vi "SwTmr Main.vi"() -> ()   [LabVIEW 2017]
doc: "This sample project is built upon the standard state machine template and shows how you could create an application that acquires, analyzes, and presents data. It includes functionality for presenting configuration dialogs, preserving settings between executions, loading and saving data, as well as exporting graph images and text files.\n\nIt is most appropriate for data that is acquired instantly as it does not allow for screen updates mid acquisition nor does it allow for continuous streaming to disk."
uses:
  controls/SwTmr State.ctl
  controls/SwTmr Data.ctl
  controls/SwTmr UI References.ctl
  controls/SwTmr Graph Data.ctl
  <vilib>/Utility/miscctls.llb/LVAnnotationListTypeDef.ctl
  <vilib>/Utility/miscctls.llb/LVCursorListTypeDef.ctl
  controls/SwTmr User Specified Data.ctl
  controls/SwTmr HW Configuration.ctl
  controls/SwTmr Analysis Configuration.ctl
  controls/SwTmr New Data Behavior.ctl
  controls/SwTmr Transfer Func File Path.ctl
  <vilib>/Utility/file.llb/Read Delimited Spreadsheet (DBL).vi
panel:
  in  "Settings":bool
  in  "Snapshot":bool
  in  "Analyze":bool
  in  "Clear":bool
  in  "Exit":bool
  in  "Acquire":bool
  in  "Export":bool
  in  "Save Data":bool
  in  "Load Data":bool
  out "Ch4 Error (mm:ss)":dbl format="%<%M:%S>t"
  out "Ch3 Error (mm:ss)":dbl format="%<%M:%S>t"
  out "Ch2 Error (mm:ss)":dbl format="%<%M:%S>t"
  out "Ch1 Error (mm:ss)":dbl format="%<%M:%S>t"
  out "Ch0 Error (mm:ss)":dbl format="%<%M:%S>t"
  out "Ch4 Time (mm:ss)":dbl format="%<%M:%S>t"
  out "Ch3 Time (mm:ss)":dbl format="%<%M:%S>t"
  out "Ch2 Time (mm:ss)":dbl format="%<%M:%S>t"
  out "Ch1 Time (mm:ss)":dbl format="%<%M:%S>t"
  out "Ch0 Time (mm:ss)":dbl format="%<%M:%S>t"
  out "Raw Data Graph":waveform(dbl)[](graph)
  out "Status Bar":string
  # "ROGERS RESEARCH GROUP"
  # "Electrochemical Stopwatch Readout System"
  # "+/-"
  # "+/-"
  # "+/-"
  # "+/-"
  # "+/-"
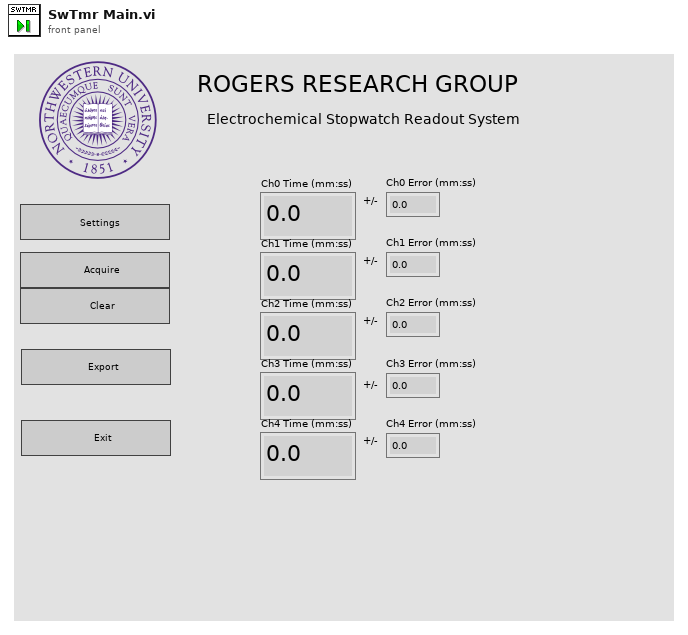
[diagram p1: front panel]
types:
  T1 = typedef "SwTmr Data.ctl" = cluster{"UI References":T2, "Graph Data":T3, "User Specified":T6}
  T2 = typedef "SwTmr UI References.ctl" = cluster{"Stop Ref":refnum<vi>, "Save Ref":refnum<vi>, "Open Ref":refnum<vi>, "Export Ref":refnum<vi>, "Acquire Ref":refnum<vi>, "Configure Ref":refnum<vi>, "Graph Ref":refnum<vi>, "Clear Ref":refnum<vi>, "Analyze Ref":refnum<vi>, "Status Ref":refnum<vi>, "Snapshot Ref":refnum<vi>}
  T3 = typedef "SwTmr Graph Data.ctl" = cluster{"Data":waveform(dbl)[], "Annotation List":T4, "Cursor List":T5, "Analysis Data":waveform(dbl)[]}
  T4 = typedef "LVAnnotationListTypeDef.ctl" = cluster{"Name":string, "Color":u32, "Style":u8, "Point Style":u8, "Name Visible":bool, "Allow Drag":bool, "Annotation Mode":u32, "Plot":i32, "Index":i32, "Position":cluster{"X":dbl, "Y":dbl}, "X Scale":u32, "Y Scale":u32, "Show Arrow":bool, "Lock Name":bool, "Plot Area":i32, "Label Offset":cluster{"X":dbl, "Y":dbl}}[]
  T5 = typedef "LVCursorListTypeDef.ctl" = cluster{"Name":string, "Color":u32, "Style":u8, "Point Style":u8, "Name Visible":bool, "Allow Drag":bool, "Cursor Mode":u32, "Plot":i32, "Index":i32, "Position":cluster{"X":dbl, "Y":dbl}, "X Scale":u32, "Y Scale":u32, "Watch Plots":i32[], "Watch All Plots":bool, "Plot Area":i32, "Label Offset":cluster{"X":dbl, "Y":dbl}}[]
  T6 = typedef "SwTmr User Specified Data.ctl" = cluster{"Hardware Configuration":T7, "Analysis Configuration":T8, "New Data Behavior":T9, "Time-Voltage transfer function file path (dialog if empty)":T10, "Cell (V) Error Upper":dbl, "Cell (V) Error Lower (type \"-\")":dbl}
  T7 = typedef "SwTmr HW Configuration.ctl" = cluster{"Physical Channel":tag, "Maximum Input":dbl, "Minimum Input":dbl, "Sample Rate":dbl, "Number of Samples":i32}
  T8 = typedef "SwTmr Analysis Configuration.ctl" = cluster{"Statistics":bool}
  T9 = typedef "SwTmr New Data Behavior.ctl" = enum16{"Replace", "Overlay", "Append"}
  T10 = typedef "SwTmr Transfer Func File Path.ctl" = path
  T11 = typedef "SwTmr State.ctl" = enum16{"Initialize", "Wait for Event", "Update UI", "Configure", "Acquire", "Load Data", "Save Data", "Clear Data", "Export Data", "Analyze", "Copy Graph", "Exit"}
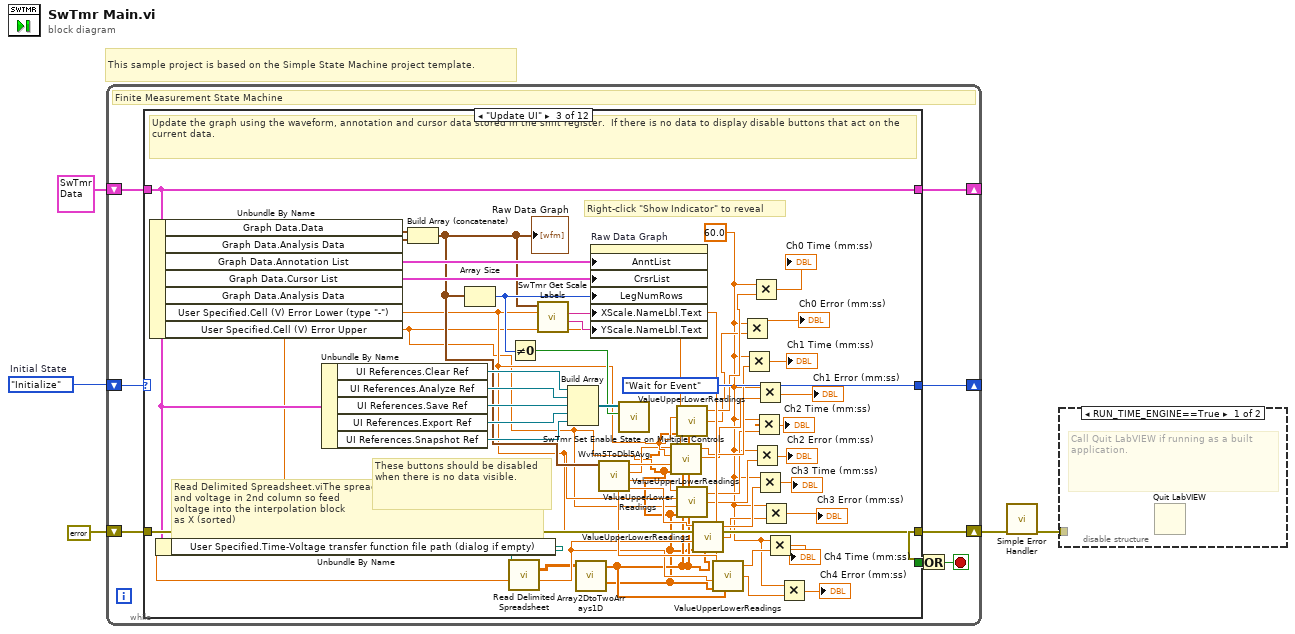
[diagram p0: block diagram]
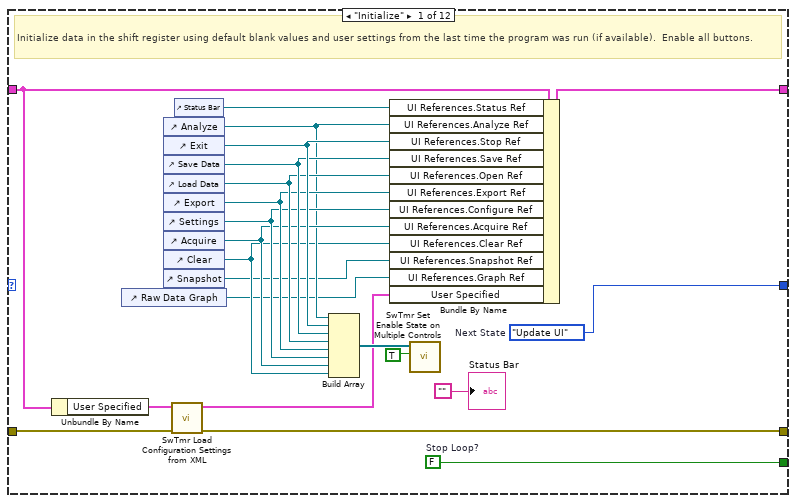
[diagram p3: hidden frame]
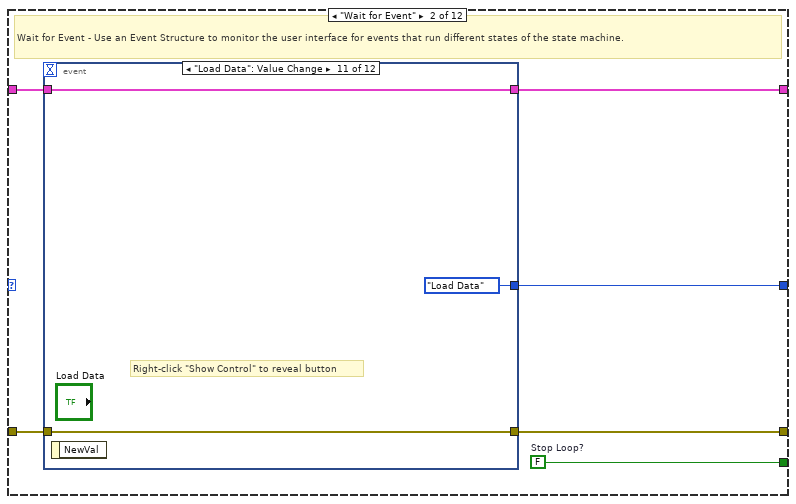
[diagram p4: hidden frame]
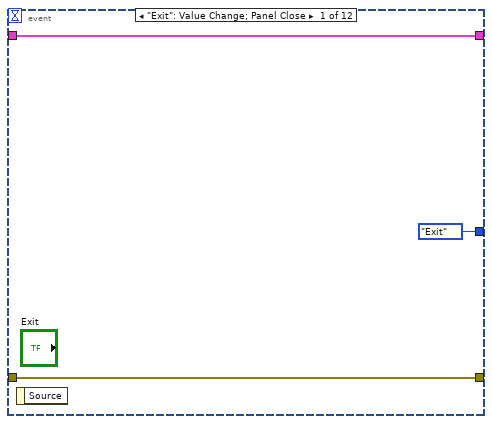
[diagram p5: hidden frame]
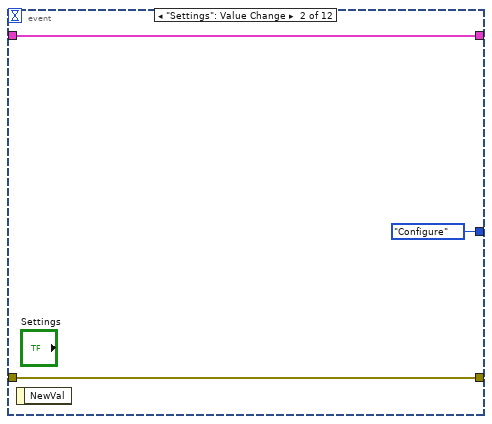
[diagram p6: hidden frame]
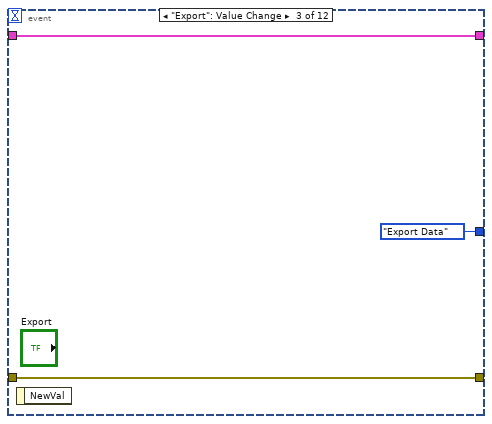
[diagram p7: hidden frame]
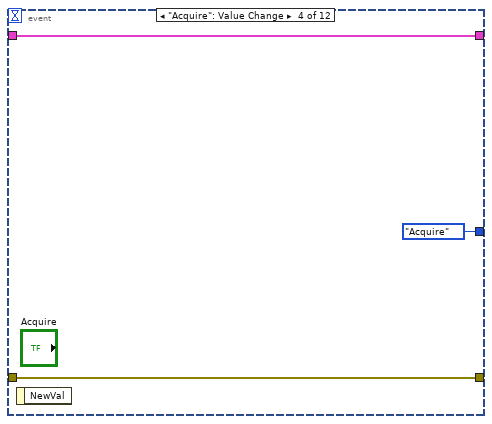
[diagram p8: hidden frame]
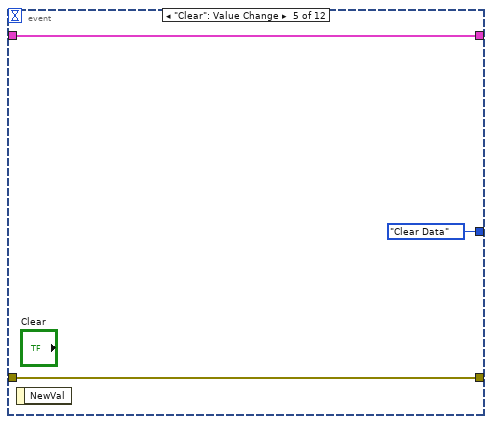
[diagram p9: hidden frame]
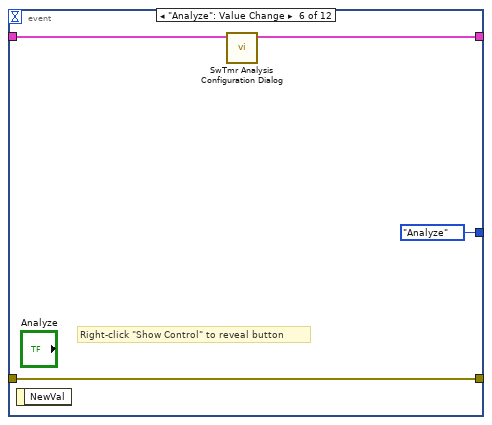
[diagram p10: hidden frame]
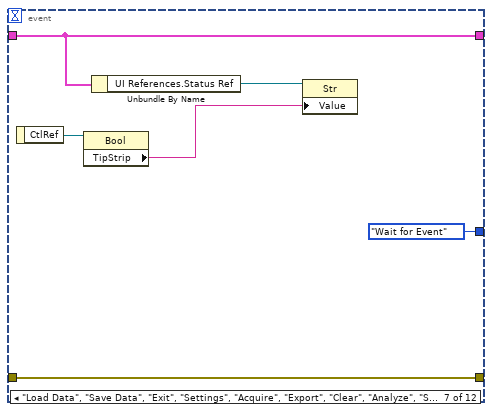
[diagram p11: hidden frame]
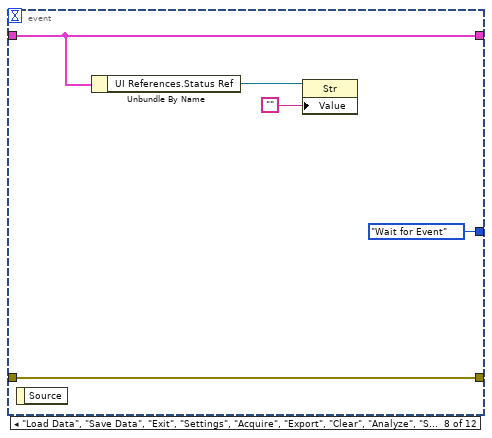
[diagram p12: hidden frame]
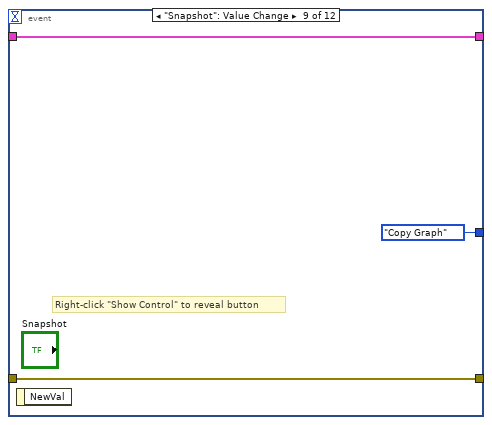
[diagram p13: hidden frame]
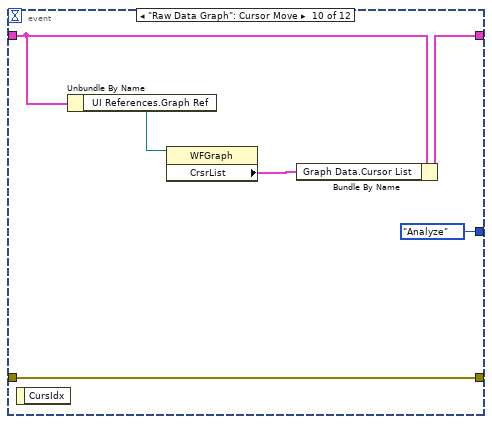
[diagram p14: hidden frame]
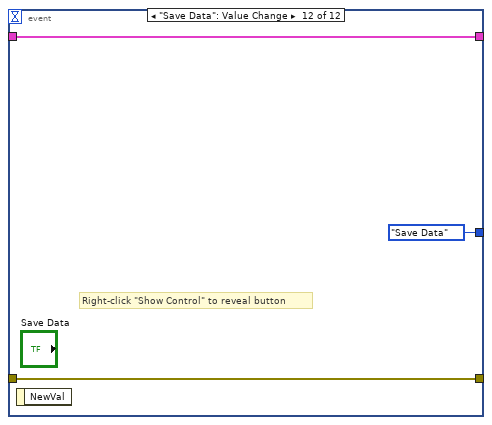
[diagram p15: hidden frame]
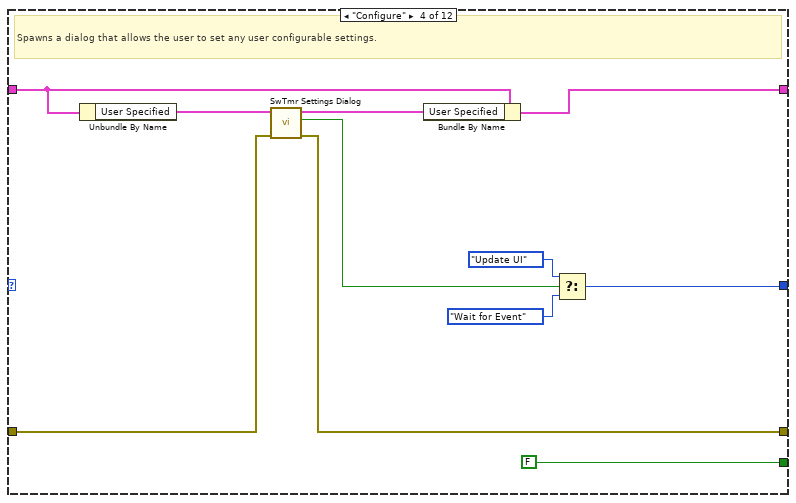
[diagram p16: hidden frame]
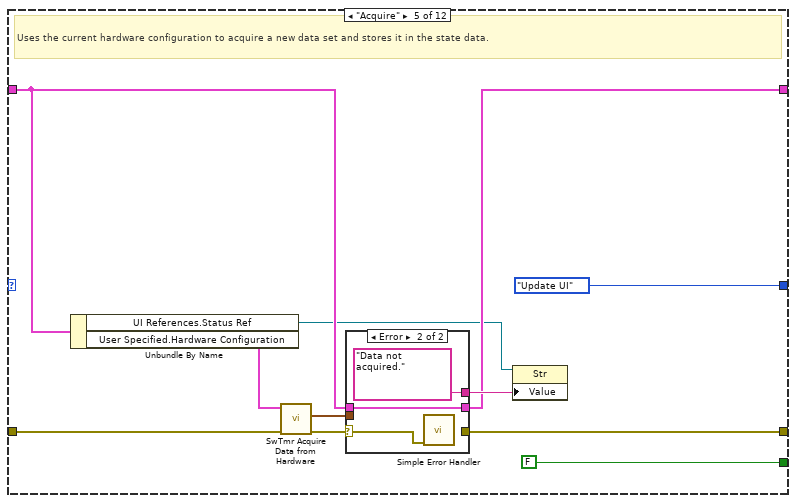
[diagram p17: hidden frame]
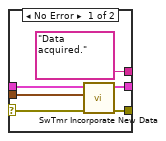
[diagram p18: hidden frame]
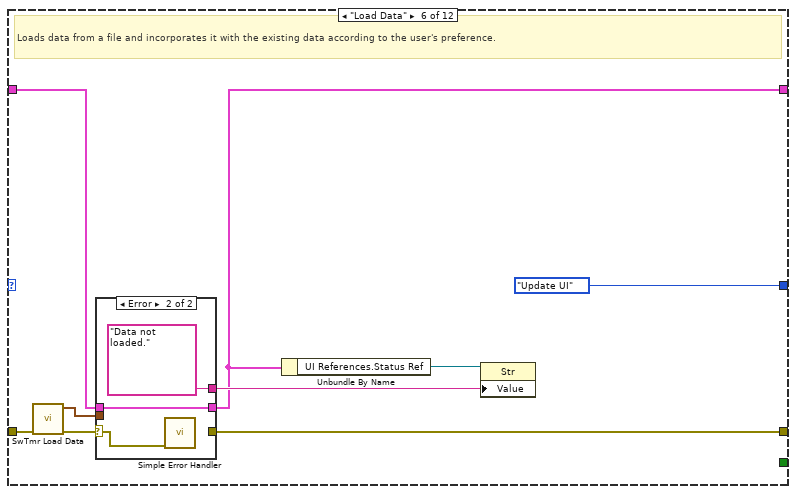
[diagram p19: hidden frame]
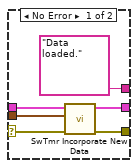
[diagram p20: hidden frame]
diagram:
  w5 = SwTmr_State."Initialize"  # Initial State
  # "This sample project is based on the Simple State Machine project template."
  n1 = while {
    shift-right: [w12] -> _
    shift-left: w5 -> [w13]
    shift-right: [w10] -> _
    shift-left: T1 {"UI References"={"Stop Ref"=refnum, "Save Ref"=refnum, "Open Ref"=refnum, "Export Ref"=refnum, "Acquire Ref"=refnum, "Configure Ref"=refnum, "Graph Ref"=refnum, "Clear Ref"=refnum, "Analyze Ref"=refnum, "Status Ref"=refnum, "Snapshot Ref"=refnum}, "Graph Data"={"Data"=[], "Annotation List"=[], "Cursor List"=[], "Analysis Data"=[]}, "User Specified"={"Hardware Configuration"={"Physical Channel"="", "Maximum Input"=0.0, "Minimum Input"=0.0, "Sample Rate"=0.0, "Number of Samples"=0}, "Analysis Configuration"={"Statistics"=FALSE}, "New Data Behavior"=enum."Replace", "Time-Voltage transfer function file path (dialog if empty)"=path "", "Cell (V) Error Upper"=0.0, "Cell (V) Error Lower (type \"-\")"=0.0}} ("Data") -> [w11]
    shift-right: [w6] -> w2
    shift-left: errorcluster {"status"=FALSE, "code"=0, "source"=""} ("error constant") -> [w9]
    stop <- w7 stop-if-true
    # "Finite Measurement State Machine"
    n2 = case shown="\"Update UI\"" w13 {
      tunnel: [w35 w41 SwTmr_State."Wait for Event" ("(Value Not Used)") w140 SwTmr_State."Update UI" ("Next State") SwTmr_State."Update UI" ("(Value Not Used)") SwTmr_State."Wait for Event" ("(Value Not Used)") SwTmr_State."Wait for Event" ("(Value Not Used)") SwTmr_State."Update UI" ("(Value Not Used)") SwTmr_State."Update UI" ("(Value Not Used)") SwTmr_State."Wait for Event" ("(Value Not Used)") w230] -> w12
      tunnel: [w34 w40 _ FALSE ("Stop Loop?") FALSE ("Stop Loop?") _ _ _ _ _ _ w229] -> w8
      tunnel: w11 -> [w25 w39 w119 w146 w153 w176 w189 w201 w212 w215 w221 w227]
      tunnel: [w33 w38 w119 w145 w152 w170 w189 w201 w211 w215 w221 w227] -> w10
      tunnel: w9 -> [w23 w37 w136 w144 w155 w175 w191 w204 w214 w217 w220 w224]
      tunnel: [w22 w36 w136 w143 w148 w174 w187 w198 w214 w217 w219 w223] -> w6
      frame "Initialize" {
        w34 = FALSE  # Stop Loop?
        w35 = SwTmr_State."Update UI"  # Next State
        # "Initialize data in the shift register using default blank values and user settings from the last time the program was run (if available).  Enable all buttons."
        n3 = Unbundle By Name(w25) -> ("User Specified"=w24:T6)
        n4 = control-ref of="Raw Data Graph"() -> (w14:refnum<vi>)
        n5 = control-ref of="Analyze"() -> (w21:refnum<vi>)
        n6 = control-ref of="Exit"() -> (w32:refnum<vi>)
        n7 = control-ref of="Save Data"() -> (w31:refnum<vi>)
        n8 = control-ref of="Load Data"() -> (w30:refnum<vi>)
        n9 = control-ref of="Export"() -> (w29:refnum<vi>)
        n10 = control-ref of="Settings"() -> (w28:refnum<vi>)
        n11 = control-ref of="Acquire"() -> (w27:refnum<vi>)
        n12 = control-ref of="Clear"() -> (w19:refnum<vi>)
        n13 = control-ref of="Snapshot"() -> (w15:refnum<vi>)
        n14 = call "SwTmr Load Configuration Settings from XML.vi"("error in (no error)"=w23, "User Configuration in"=w24) -> ("error out"=w22:errorcluster, "User Configuration out"=w17:T6)  [unwired: 8 in]
        n15 = control-ref of="Status Bar"() -> (w20:refnum<vi>)
        n16 = Build Array(w21, w32, w31, w30, w29, w28, w27, w19) -> (w26:refnum<vi>[])
        n17 = Bundle By Name(cluster=w25, "UI References.Status Ref"=w20, "UI References.Analyze Ref"=w21, "UI References.Stop Ref"=w32, "UI References.Save Ref"=w31, "UI References.Open Ref"=w30, "UI References.Export Ref"=w29, "UI References.Configure Ref"=w28, "UI References.Acquire Ref"=w27, "UI References.Clear Ref"=w19, "UI References.Snapshot Ref"=w15, "UI References.Graph Ref"=w14, "User Specified"=w17) -> (w33:T1)
        n18 = call "SwTmr Set Enable State on Multiple Controls.vi"("Enable?"=TRUE, "Controls"=w26) -> ()  [unwired: 10 in]
        "Status Bar" <- "" ("Status Bar")
      }
      frame "Wait for Event" {
        w40 = FALSE  # Stop Loop?
        # "Wait for Event - Use an Event Structure to monitor the user interface for events that run different states of the state machine."
        n19 = event shown="[10] \"Load Data\": Value Change" {
          selector: _ -> [_ _ _ _ _ _ _ _ _ _ _ _]
          dyn-events: _ -> [_ _ _ _ _ _ _ _ _ _ _ _]
          timeout: _ -> [_ _ _ _ _ _ _ _ _ _ _ _]
          tunnel: [SwTmr_State."Exit" ("Next State") SwTmr_State."Configure" ("Next State") SwTmr_State."Export Data" ("Next State") SwTmr_State."Acquire" ("Next State") SwTmr_State."Clear Data" ("Next State") SwTmr_State."Analyze" ("Next State") SwTmr_State."Wait for Event" ("Next State") SwTmr_State."Wait for Event" ("Next State") SwTmr_State."Copy Graph" ("Next State") SwTmr_State."Analyze" ("Next State") SwTmr_State."Load Data" ("Next State") SwTmr_State."Save Data" ("Next State")] -> w41
          tunnel: w39 -> [w43 w47 w50 w53 w56 w58 w64 w70 w74 w75 w82 w85]
          tunnel: [w43 w47 w50 w53 w56 w57 w64 w70 w74 w78 w82 w85] -> w38
          tunnel: w37 -> [w42 w46 w49 w52 w55 w60 w66 w71 w73 w80 w81 w84]
          tunnel: [w42 w46 w49 w52 w55 w60 w66 w71 w73 w80 w81 w84] -> w36
          event "Exit": Value Change; Panel Close {
            n20 = event-data() -> ()  [unwired: 1 in, 1 out]
          }
          event "Settings": Value Change {
            n21 = event-data() -> ()  [unwired: 1 in, 1 out]
          }
          event "Export": Value Change {
            n22 = event-data() -> ()  [unwired: 1 in, 1 out]
          }
          event "Acquire": Value Change {
            n23 = event-data() -> ()  [unwired: 1 in, 1 out]
          }
          event "Clear": Value Change {
            n24 = event-data() -> ()  [unwired: 1 in, 1 out]
          }
          event "Analyze": Value Change {
            # "Right-click \"Show Control\" to reveal button"
            n25 = event-data() -> ()  [unwired: 1 in, 1 out]
            n26 = call "SwTmr Analysis Configuration Dialog.vi"("Data in"=w58) -> ("Data out"=w57:T1)  [unwired: 10 in]
          }
          event "Load Data", "Save Data", "Exit", "Settings", "Acquire", "Export", "Clear", "Analyze", "Snapshot": Mouse Enter {
            n27 = event-data() -> ("CtlRef"=w65:refnum<vi>)  [unwired: 1 in]
            n28 = property class="Bool"(reference=w65) -> ("TipStrip"=w62:string)  [unwired: 1 in, 2 out]
            n29 = Unbundle By Name(w64) -> ("UI References.Status Ref"=w63:refnum<vi>)
            n30 = property class="Str"(reference=w63, "Value"=w62) -> ()  [unwired: 1 in, 2 out]
          }
          event "Load Data", "Save Data", "Exit", "Settings", "Acquire", "Export", "Clear", "Analyze", "Snapshot": Mouse Leave {
            n31 = event-data() -> ()  [unwired: 1 in, 1 out]
            n32 = Unbundle By Name(w70) -> ("UI References.Status Ref"=w69:refnum<vi>)
            n33 = property class="Str"(reference=w69, "Value"="") -> ()  [unwired: 1 in, 2 out]
          }
          event "Snapshot": Value Change {
            # "Right-click \"Show Control\" to reveal button"
            n34 = event-data() -> ()  [unwired: 1 in, 1 out]
          }
          event "Raw Data Graph": Cursor Move {
            n35 = event-data() -> ()  [unwired: 1 in, 1 out]
            n36 = Unbundle By Name(w75) -> ("UI References.Graph Ref"=w77:refnum<vi>)
            n37 = property class="WFGraph"(reference=w77) -> ("CrsrList"=w76:T5)  [unwired: 1 in, 2 out]
            n38 = Bundle By Name(cluster=w75, "Graph Data.Cursor List"=w76) -> (w78:T1)
          }
          event "Load Data": Value Change {
            # "Right-click \"Show Control\" to reveal button"
            n39 = event-data() -> ()  [unwired: 1 in, 1 out]
          }
          event "Save Data": Value Change {
            # "Right-click \"Show Control\" to reveal button"
            n40 = event-data() -> ()  [unwired: 1 in, 1 out]
          }
        }
      }
      frame "Update UI" {
        w88 = 60.0 ("x")
        # "Right-click \"Show Indicator\" to reveal"
        # "Read Delimited Spreadsheet.viThe spreadsheet has time in 1st column\nand voltage in 2nd column so feed\nvoltage into the interpolation block\nas X (sorted)"
        # "These buttons should be disabled when there is no data visible."
        # "Update the graph using the waveform, annotation and cursor data stored in the shift register.  If there is no data to display disable buttons that act on the current data."
        n41 = Unbundle By Name(w119) -> ("Graph Data.Data"=w130:waveform(dbl)[], "Graph Data.Analysis Data"=w121:waveform(dbl)[], "Graph Data.Annotation List"=w134:T4, "Graph Data.Cursor List"=w131:T5, "User Specified.Cell (V) Error Lower (type \"-\")"=w117:dbl, "User Specified.Cell (V) Error Upper"=w112:dbl)  [unwired: 1 out]
        n42 = Unbundle By Name(w119) -> ("User Specified.Time-Voltage transfer function file path (dialog if empty)"=w109:T10)
        n43 = Unbundle By Name(w119) -> ("UI References.Clear Ref"=w127:refnum<vi>, "UI References.Analyze Ref"=w126:refnum<vi>, "UI References.Save Ref"=w133:refnum<vi>, "UI References.Export Ref"=w124:refnum<vi>, "UI References.Snapshot Ref"=w125:refnum<vi>)
        n44 = Build Array (concatenate)(w130, w121) -> (w120:waveform(dbl)[])
        "Raw Data Graph" <- w120
        n45 = Array Size(array=w120) -> (size(s)=w129:i32)
        n46 = call-poly <vilib>:"Read Delimited Spreadsheet.vi"("file path (dialog if empty)"=w109) -> ("all rows"=w108:dbl[][])  [unwired: 9 in, 5 out]
        n47 = Not Equal To 0?(x=w129) -> (x != 0?=w128:bool)
        n48 = call "SwTmr Get Scale Labels.vi"("Array of Waveforms"=w120) -> ("Y Scale Label Text"=w122:string, "X Scale Label Text"=w123:string)  [unwired: 9 in]
        n49 = Build Array(w127, w126, w133, w124, w125) -> (w132:refnum<vi>[])
        n50 = call "Array2DtoTwoArrays1D.vi"("Input (2D array)"=w108) -> ("Y Data Array"=w110:dbl[], "X Data Array"=w111:dbl[])  [unwired: 2 in]
        n51 = property on="Raw Data Graph" class="WFGraph (strict)"("AnntList"=w134, "CrsrList"=w131, "LegNumRows"=w129, "XScale.NameLbl.Text"=w123, "YScale.NameLbl.Text"=w122) -> ()  [unwired: 2 in, 2 out]
        n52 = call "Wvfm5ToDbl5Avg.vi"("Wvfm"=w120) -> ("Ch3Avg"=w116:dbl, "Ch2Avg"=w113:dbl, "Ch1Avg"=w114:dbl, "Ch0Avg"=w115:dbl, "Ch4Avg"=w118:dbl)  [unwired: 6 in]
        n53 = call "SwTmr Set Enable State on Multiple Controls.vi"("Enable?"=w128, "Controls"=w132) -> ()  [unwired: 10 in]
        n54 = call "ValueUpperLowerReadings.vi"("Target Value"=w114, "Lower X Error Value (type -0.01 for neg 10mV)"=w117, "Upper X Error Value (type 0.01 for pos 10mV)"=w112, "X Data (sorted)"=w110, "Y Data"=w111) -> ("Interpolated Result"=w105:dbl, "Error"=w95:dbl)  [unwired: 1 in]
        n55 = call "ValueUpperLowerReadings.vi"("Target Value"=w115, "Lower X Error Value (type -0.01 for neg 10mV)"=w117, "Upper X Error Value (type 0.01 for pos 10mV)"=w112, "X Data (sorted)"=w110, "Y Data"=w111) -> ("Interpolated Result"=w107:dbl, "Error"=w97:dbl)  [unwired: 1 in]
        n56 = call "ValueUpperLowerReadings.vi"("Target Value"=w113, "Lower X Error Value (type -0.01 for neg 10mV)"=w117, "Upper X Error Value (type 0.01 for pos 10mV)"=w112, "X Data (sorted)"=w110, "Y Data"=w111) -> ("Interpolated Result"=w103:dbl, "Error"=w92:dbl)  [unwired: 1 in]
        n57 = call "ValueUpperLowerReadings.vi"("Target Value"=w116, "Lower X Error Value (type -0.01 for neg 10mV)"=w117, "Upper X Error Value (type 0.01 for pos 10mV)"=w112, "X Data (sorted)"=w110, "Y Data"=w111) -> ("Interpolated Result"=w102:dbl, "Error"=w90:dbl)  [unwired: 1 in]
        n58 = call "ValueUpperLowerReadings.vi"("Target Value"=w118, "Lower X Error Value (type -0.01 for neg 10mV)"=w117, "Upper X Error Value (type 0.01 for pos 10mV)"=w112, "X Data (sorted)"=w110, "Y Data"=w111) -> ("Interpolated Result"=w101:dbl, "Error"=w87:dbl)  [unwired: 1 in]
        n59 = Multiply(x=w88, y=w97) -> (x*y=→"Ch0 Error (mm:ss)":dbl)
        n60 = Multiply(x=w88, y=w105) -> (x*y=→"Ch1 Time (mm:ss)":dbl)
        n61 = Multiply(x=w88, y=w107) -> (x*y=→"Ch0 Time (mm:ss)":dbl)
        n62 = Multiply(x=w88, y=w92) -> (x*y=→"Ch2 Error (mm:ss)":dbl)
        n63 = Multiply(x=w88, y=w103) -> (x*y=→"Ch2 Time (mm:ss)":dbl)
        n64 = Multiply(x=w88, y=w95) -> (x*y=→"Ch1 Error (mm:ss)":dbl)
        n65 = Multiply(x=w88, y=w102) -> (x*y=→"Ch3 Time (mm:ss)":dbl)
        n66 = Multiply(x=w88, y=w90) -> (x*y=→"Ch3 Error (mm:ss)":dbl)
        n67 = Multiply(x=w88, y=w101) -> (x*y=→"Ch4 Time (mm:ss)":dbl)
        n68 = Multiply(x=w88, y=w87) -> (x*y=→"Ch4 Error (mm:ss)":dbl)
      }
      frame "Configure" {
        # "Spawns a dialog that allows the user to set any user configurable settings."
        n69 = Unbundle By Name(w146) -> ("User Specified"=w138:T6)
        n70 = call "SwTmr Settings Dialog.vi"("error in (no error)"=w144, "Configuration in"=w138) -> ("error out"=w143:errorcluster, "UI Refresh Needed?"=w142:bool, "Configuration out"=w137:T6)  [unwired: 7 in]
        n71 = Bundle By Name(cluster=w146, "User Specified"=w137) -> (w145:T1)
        n72 = Select(t=SwTmr_State."Update UI" ("Next State if true"), s=w142, f=SwTmr_State."Wait for Event" ("Next State if false")) -> (s? t:f=w140:T11)
      }
      frame "Acquire" {
        # "Uses the current hardware configuration to acquire a new data set and stores it in the state data."
        n73 = Unbundle By Name(w153) -> ("UI References.Status Ref"=w149:refnum<vi>, "User Specified.Hardware Configuration"=w156:T7)
        n74 = call "SwTmr Acquire Data from Hardware.vi"("error in (no error)"=w155, "Hardware Configuration"=w156) -> ("error out"=w150:errorcluster, "Graph Data"=w151:waveform(dbl)[])  [unwired: 7 in]
        n75 = case shown="Error" w150 {
          selector: w150 -> [w161 w166]
          tunnel: w153 -> [w160 w167]
          tunnel: [w164 w167] -> w152
          tunnel: [w163 _] -> w148
          tunnel: w151 -> [w162 _]
          tunnel: ["Data acquired." ("Data acquired") "Data not acquired." ("Data not acquired")] -> w154
          frame No Error {
            n76 = call "SwTmr Incorporate New Data.vi"("error in (no error)"=w161, "New Graph Data"=w162, "Data in"=w160) -> ("error out"=w163:errorcluster, "Data out"=w164:T1)  [unwired: 7 in]
          }
          frame Error {
            n77 = call <vilib>:"Simple Error Handler.vi"("error in (no error)"=w166) -> ()  [unwired: 4 in, 5 out]
          }
        }
        n78 = property class="Str"(reference=w149, "Value"=w154) -> ()  [unwired: 1 in, 2 out]
      }
      frame "Load Data" {
        # "Loads data from a file and incorporates it with the existing data according to the user's preference."
        n79 = call "SwTmr Load Data.vi"("error in (no error)"=w175) -> ("error out"=w172:errorcluster, "New Graph Data"=w169:waveform(dbl)[])  [unwired: 9 in]
        n80 = case shown="Error" w172 {
          selector: w172 -> [w179 w184]
          tunnel: w176 -> [w178 w185]
          tunnel: [w182 w185] -> w170
          tunnel: [w181 _] -> w174
          tunnel: w169 -> [w180 _]
          tunnel: ["Data loaded." ("Data loaded") "Data not loaded." ("Data not loaded")] -> w171
          frame No Error {
            n81 = call "SwTmr Incorporate New Data.vi"("error in (no error)"=w179, "New Graph Data"=w180, "Data in"=w178) -> ("error out"=w181:errorcluster, "Data out"=w182:T1)  [unwired: 7 in]
          }
          frame Error {
            n82 = call <vilib>:"Simple Error Handler.vi"("error in (no error)"=w184) -> ()  [unwired: 4 in, 5 out]
          }
        }
        n83 = Unbundle By Name(w170) -> ("UI References.Status Ref"=w168:refnum<vi>)
        n84 = property class="Str"(reference=w168, "Value"=w171) -> ()  [unwired: 1 in, 2 out]
      }
      frame "Save Data" {
        # "Saves the existing measurement data to a file."
        n85 = Unbundle By Name(w189) -> ("UI References.Status Ref"=w188:refnum<vi>, "Graph Data.Data"=w192:waveform(dbl)[])
        n86 = call "SwTmr Save Data.vi"("error in (no error)"=w191, "Data"=w192) -> ("error out"=w190:errorcluster)  [unwired: 9 in]
        n87 = case shown="No Error" w190 {
          selector: w190 -> [w194 w197]
          tunnel: ["Data saved." ("Data saved") "Data not saved." ("Data not saved")] -> w186
          tunnel: [w194 _] -> w187
          frame No Error {
          }
          frame Error {
            n88 = call <vilib>:"Simple Error Handler.vi"("error in (no error)"=w197) -> ()  [unwired: 4 in, 5 out]
          }
        }
        n89 = property class="Str"(reference=w188, "Value"=w186) -> ()  [unwired: 1 in, 2 out]
      }
      frame "Export Data" {
        # "Exports the currently loaded measurement and analysis data to a text file that can be imported into a spreadsheet or other application."
        n90 = Unbundle By Name(w201) -> ("UI References.Status Ref"=w199:refnum<vi>, "Graph Data"=w200:T3)
        n91 = call "SwTmr Export Data.vi"("error in (no error)"=w204, "Graph Data"=w200) -> ("error out"=w202:errorcluster)  [unwired: 9 in]
        n92 = case shown="Error" w202 {
          selector: w202 -> [w206 w209]
          tunnel: ["Data exported." ("Data exported") "Data not exported." ("Data not exported")] -> w203
          tunnel: [w206 _] -> w198
          frame No Error {
          }
          frame Error {
            n93 = call <vilib>:"Simple Error Handler.vi"("error in (no error)"=w209) -> ()  [unwired: 4 in, 5 out]
          }
        }
        n94 = property class="Str"(reference=w199, "Value"=w203) -> ()  [unwired: 1 in, 2 out]
      }
      frame "Clear Data" {
        # "Clears the data currently in the graph."
        n95 = Bundle By Name(cluster=w212, "Graph Data"=T3 {"Data"=[], "Annotation List"=[], "Cursor List"=[], "Analysis Data"=[]} ("Graph")) -> (w211:T1)
      }
      frame "Analyze" {
        # "#CodeRecommended - add your own signal analysis here."
        # "Analyzes the measurement data using the user selected routines and adds annotations and calculated channels to the graph where appropriate."
        n96 = Unbundle By Name(w215) -> ("Graph Data"=w216:T3)
        n97 = call "SwTmr Statistical Analysis.vi"("Graph Data In"=w216) -> ()  [unwired: 8 in, 2 out]
      }
      frame "Copy Graph" {
        # "Places an image of the graph on the clipboard for pasting into reports or emails."
        n98 = call "SwTmr Copy Graph to Clipboard.vi"("error in (no error)"=w220, "Graph Data"=w221) -> ("error out"=w219:errorcluster)  [unwired: 9 in]
      }
      frame "Exit" {
        w229 = TRUE  # Stop Loop?
        w230 = SwTmr_State."Exit"  # (Value Not Used)
        # "The state value is not used here since this is the last iteration of the state machine loop"
        # "Saves the user's settings to an XML file and stops execution."
        n99 = Unbundle By Name(w227) -> ("UI References.Status Ref"=w225:refnum<vi>, "User Specified"=w228:T6)
        n100 = call "SwTmr Save Configuration Settings to XML.vi"("error in (no error)"=w224, "User Configuration"=w228) -> ("error out"=w223:errorcluster)  [unwired: 9 in]
        n101 = property class="Str"(reference=w225, "Value"="Stopped." ("Stopped")) -> ()  [unwired: 1 in, 2 out]
      }
    }
    n102 = Or(x=w6, y=w8) -> (x .or. y?=w7:bool)
  }
  n103 = call <vilib>:"Simple Error Handler.vi"("error in (no error)"=w2) -> ("error out"=w1:errorcluster)  [unwired: 4 in, 4 out]
  n104 = disable-structure shown="RUN_TIME_ENGINE==True" {
    disable-tunnel: w1 -> [_ _]
    frame condition #0 {
      # "Call Quit LabVIEW if running as a built application."
      n105 = Quit LabVIEW() -> ()  [unwired: 1 in]
    }
    frame condition #1 (active) {
    }
  }
